vi "CIC 8192 IQx1.vi"(0 "data":T1, 1 "reset":bool, 5 "config":cluster{"factor":fxp<+,16,16>, "shift":i16}, 7 "config valid":bool, 9 "input valid":bool) -> (4 "i out":fxp<+/-,64,1>, 6 "q out":fxp<+/-,64,1>, 10 "output valid":bool)   [LabVIEW 2017, in "Lock-In Amplifier Example FPGA.lvlib"]
uses:
  Lock-In Amplifier Example FPGA.lvlib
  <instrlib>/_niInstr/DSP/v1/Shared/Public/IQ Data.ctl
  <instrlib>/_niInstr/DSP/v1/Shared/niInstr DSP v1 Shared.lvlib
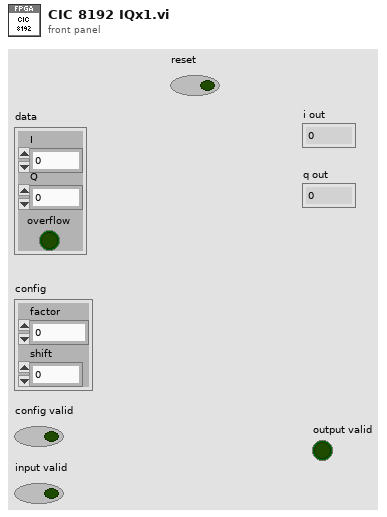
[diagram p1: front panel]
types:
  T1 = typedef "niInstr DSP v1 Shared.lvlib/IQ Data.ctl" = cluster{"I":fxp<+/-,18,1>, "Q":fxp<+/-,18,1>, "overflow":bool}
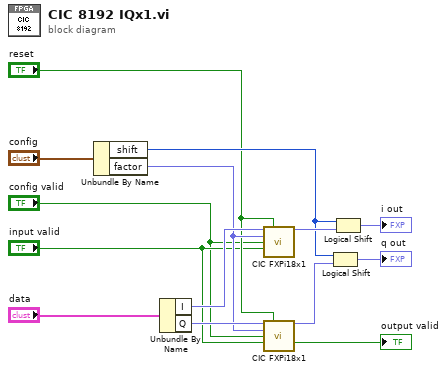
[diagram p0: block diagram]
diagram:
  n1 = Unbundle By Name("config") -> ("shift"=w8:i16, "factor"=w7:fxp<+,16,16>)
  n2 = Unbundle By Name("data") -> ("I"=w14:fxp<+/-,18,1>, "Q"=w12:fxp<+/-,18,1>)
  n3 = call "CIC FXPi18x1.vi"("input"=w14, "reset"="reset", "decimation factor"=w7, "config valid"="config valid", "input valid"="input valid") -> ("output"=w13:fxp<+,64,64>)  [unwired: 9 in, 1 out]
  n4 = call "CIC FXPi18x1.vi"("input"=w12, "reset"="reset", "decimation factor"=w7, "config valid"="config valid", "input valid"="input valid") -> ("output"=w11:fxp<+,64,64>, "output valid"=→"output valid":bool)  [unwired: 9 in]
  n5 = Logical Shift(y=w8, x=w11) -> (x << y=→"q out":fxp<+,64,64>)
  n6 = Logical Shift(y=w8, x=w13) -> (x << y=→"i out":fxp<+,64,64>)
